vi "_Raise New Window Requested.vi"(4 "WebView2.lvlib:WebView2 Control.lvclass":refnum<class "WebView2 Control.lvclass">, 5 "Event Data":cluster{"sender":refnum<k24>, "e":refnum<k24>}, 6 "Control Ref":refnum<k24>, 7 "Event Common Data":T1) -> ()   [LabVIEW 2025, in "WebView2.lvlib" / "WebView2 Control.lvclass"]
uses:
  WebView2 Control.lvclass
  E:/Labview/LV 2023/PPL/PPL Builder/Libs/LV-WebView2/Source/Libs/Microsoft.Web.WebView2.Core.dll
  Libs/Microsoft.Web.WebView2.Core.dll
  New Window Event Data.ctl
  WebView2 Control.lvclass/WebView2 Control.ctl
  WebView2 Event Filter Interface/WebView2 Event Filter Interface.lvclass
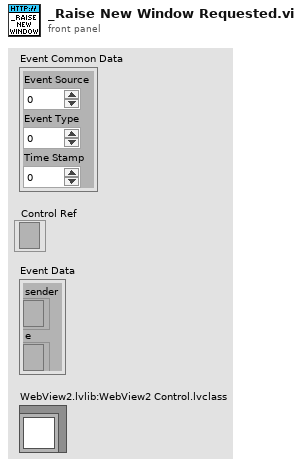
[diagram p1: front panel]
types:
  T1 = cluster{"Event Source":i32, "Event Type":u32, "Time Stamp":u32}
  T2 = typedef "WebView2.lvlib/WebView2 Control.lvclass/New Window Event Data.ctl" = cluster{"IsUserInitiated":bool, "Name":string, "Uri":string, "Filter":refnum<class "WebView2 Event Filter Interface.lvclass">, "OriginalSourceFrameInfo":refnum<k24>, "WindowFeatures":refnum<k24>}
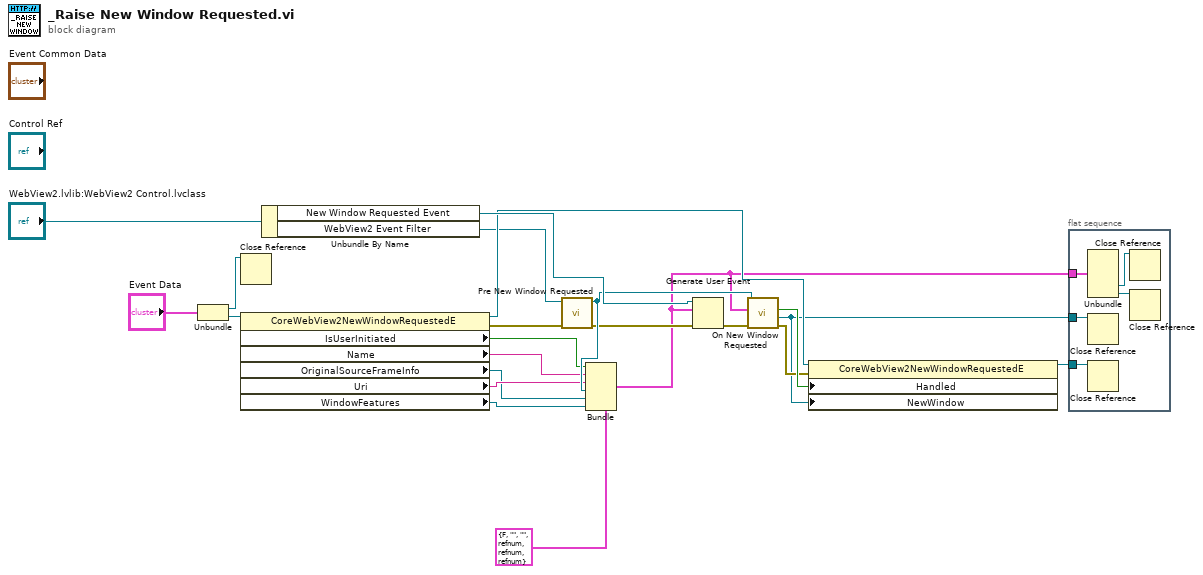
[diagram p0: block diagram]
diagram:
  n1 = Unbundle("Event Data") -> ("sender"=w15:refnum<k24>, "e"=w21:refnum<k24>)
  n2 = Close Reference(reference=w15) -> ()  [unwired: 1 in, 1 out]
  n3 = property class="CoreWebView2NewWindowRequestedE"(reference=w21) -> (reference out=w17:refnum<k24>, error out=w10:errorcluster, "IsUserInitiated"=w7:bool, "Name"=w6:string, "OriginalSourceFrameInfo"=w4:refnum<k24>, "Uri"=w5:string, "WindowFeatures"=w3:refnum<k24>)  [unwired: 1 in]
  n4 = Unbundle By Name("WebView2.lvlib:WebView2 Control.lvclass") -> ("New Window Requested Event"=w18:refnum<user-event>, "WebView2 Event Filter"=w14:refnum<class "WebView2 Event Filter Interface.lvclass">)
  n5 = call-dynamic "Pre New Window Requested.vi"("error in (no error)"=w10, "WebView2 Event Filter Interface in"=w14) -> ("error out"=w9:errorcluster, "WebView2 Event Filter Interface out"=w12:refnum<class "WebView2 Event Filter Interface.lvclass">)  [unwired: 8 in]
  n6 = Bundle(cluster=T2 {"IsUserInitiated"=FALSE, "Name"="", "Uri"="", "Filter"=refnum, "OriginalSourceFrameInfo"=refnum, "WindowFeatures"=refnum}, "IsUserInitiated"=w7, "Name"=w6, "Uri"=w5, "Filter"=w12, "OriginalSourceFrameInfo"=w4, "WindowFeatures"=w3) -> (w2:T2)
  n7 = Generate User Event(user event=w18, event data cluster=w2, error in=w9) -> (error out=w13:errorcluster)  [unwired: 1 in, 1 out]
  n8 = call-dynamic "On New Window Requested.vi"("error in (no error)"=w13, "Data"=w2, "WebView2 Event Filter Interface in"=w12) -> ("error out"=w8:errorcluster, "NewWindow"=w1:refnum<k24>, "Handled"=w11:bool)  [unwired: 6 in]
  n9 = property class="CoreWebView2NewWindowRequestedE"(reference=w17, error in=w8, "Handled"=w11, "NewWindow"=w1) -> (reference out=w16:refnum<k24>)  [unwired: 1 out]
  n10 = flat-sequence {
    tunnel: w16 -> [w27]
    tunnel: w2 -> [w26]
    tunnel: w1 -> [w25]
    frame #0 {
      n11 = Unbundle(w26) -> ("OriginalSourceFrameInfo"=w24:refnum<k24>, "WindowFeatures"=w23:refnum<k24>)  [unwired: 4 out]
      n12 = Close Reference(reference=w25) -> ()  [unwired: 1 in, 1 out]
      n13 = Close Reference(reference=w27) -> ()  [unwired: 1 in, 1 out]
      n14 = Close Reference(reference=w24) -> ()  [unwired: 1 in, 1 out]
      n15 = Close Reference(reference=w23) -> ()  [unwired: 1 in, 1 out]
    }
  }
